vi "输入框.vi"(1 "提示信息":string) -> (0 "条形码输出":string)   [LabVIEW 2020]
uses:
  Global_Variable/Global.vi
  Imm32.dll
panel:
  in  "字符串":string
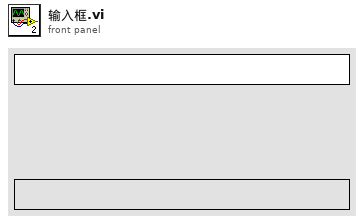
[diagram p1: front panel]
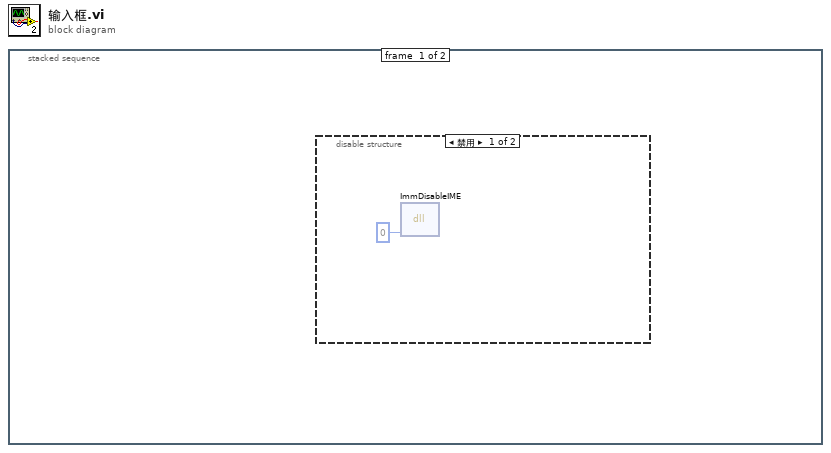
[diagram p0: block diagram]
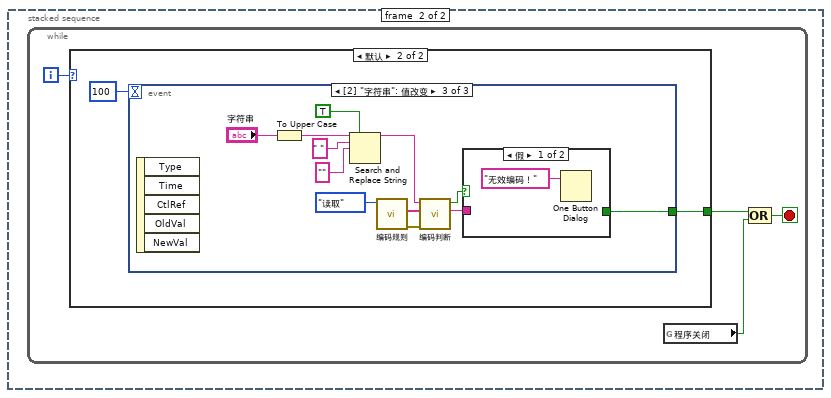
[diagram p3: hidden frame]
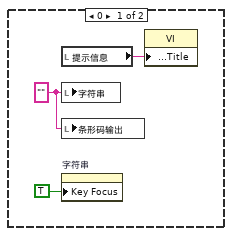
[diagram p4: hidden frame]
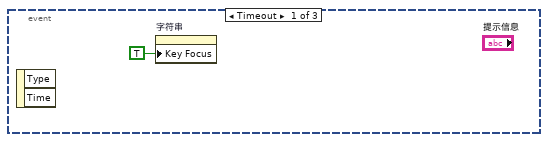
[diagram p5: hidden frame]
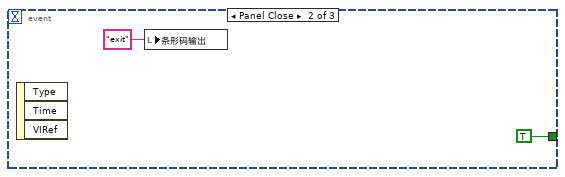
[diagram p6: hidden frame]
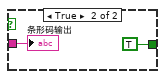
[diagram p7: hidden frame]
diagram:
  n1 = stacked-sequence {
    frame #0 {
      n2 = disable-structure shown="禁用" {
        frame Disabled {
          n3 = dll-call lib="Imm32.dll" fn="ImmDisableIME" label="SendInput"("IN"=0) -> ()  [unwired: 3 in, 4 out]
        }
        frame Enabled {
        }
      }
    }
    frame #1 {
      n4 = while {
        i -> [w4]
        stop <- w3 stop-if-true
        n5 = case shown="默认" w4 {
          tunnel: [_ w10] -> w5
          frame 0 {
            w8 = "" ("字符串")
            n6 = local read "提示信息"() -> (w7:string)
            n7 = local write "字符串"(w8) -> ()
            n8 = local write "条形码输出"(w8) -> ()
            n9 = property on="字符串" class="Str"("Key Focus"=TRUE ("键选中")) -> ()  [unwired: 2 in, 2 out]
            n10 = property class="VI"("Front Panel.Title"=w7) -> ()  [unwired: 2 in, 2 out]
          }
          frame Default {
            n11 = event shown="[2] \"字符串\": 值改变" {
              selector: _ -> [_ _ _]
              dyn-events: _ -> [_ _ _]
              timeout: 100 -> [_ _ _]
              tunnel: [_ TRUE w20] -> w10
              event Timeout {
                n12 = event-data() -> ()  [unwired: 1 in, 2 out]
                n13 = property on="字符串" class="Str"("Key Focus"=TRUE ("键选中")) -> ()  [unwired: 2 in, 2 out]
              }
              event Panel Close {
                n14 = event-data() -> ()  [unwired: 1 in, 3 out]
                n15 = local write "条形码输出"("exit" ("条形码输出")) -> ()
              }
              event "字符串": Value Change {
                n16 = event-data() -> ()  [unwired: 1 in, 5 out]
                n17 = To Upper Case(1:"字符串") -> (0:w19:string)
                n18 = Search and Replace String(replace all?=TRUE ("替换全部？(F)"), input string=w19, search string=" " ("搜索字符串"), replace string="" ("替换字符串(\"\")")) -> (result string=w14:string)  [unwired: 4 in, 3 out]
                n19 = call "编码规则.vi"("功能"=enum16{"读取", "写入"}."读取") -> ("错误输出"=w24:errorcluster, "正则表达式输出（多行）"=w25:string[])  [unwired: 8 in, 1 out]
                n20 = call "编码判断.vi"("错误输入"=w24, "编码规则"=w25, "输入编码"=w14) -> ("输出编码"=w22:string, "有效编码？"=w21:bool)  [unwired: 6 in, 1 out]
                n21 = case shown="假" w21 {
                  tunnel: w22 -> [_ w28]
                  tunnel: [_ TRUE] -> w20
                  frame False {
                    n22 = One Button Dialog(message="无效编码！" ("消息")) -> ()  [unwired: 1 in, 1 out]
                  }
                  frame True {
                    "条形码输出" <- w28
                  }
                }
              }
            }
          }
        }
        n23 = global read "Global.vi" "程序关闭"() -> (w2:bool)
        n24 = Compound Arithmetic op=OR ("复合运算")(w5, w2) -> (w3:bool)
      }
    }
  }
